vi "GenerateNewTag.vi"(8 "TagMarkerDuration (pws)":i32, 11 "Tag num":u32) -> (3 "digital waveform":digitalwaveform(waveform))   [LabVIEW 2017]
uses:
  <vilib>/Waveform/DWDTOps.llb/DWDT Boolean Array to Digital.vi
panel:
  out "Error Out":errorcluster
  in  "Error in":errorcluster
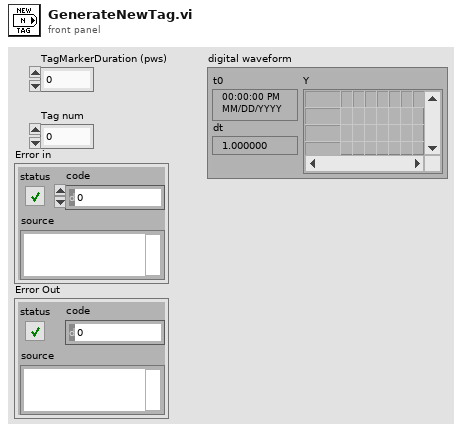
[diagram p1: front panel]
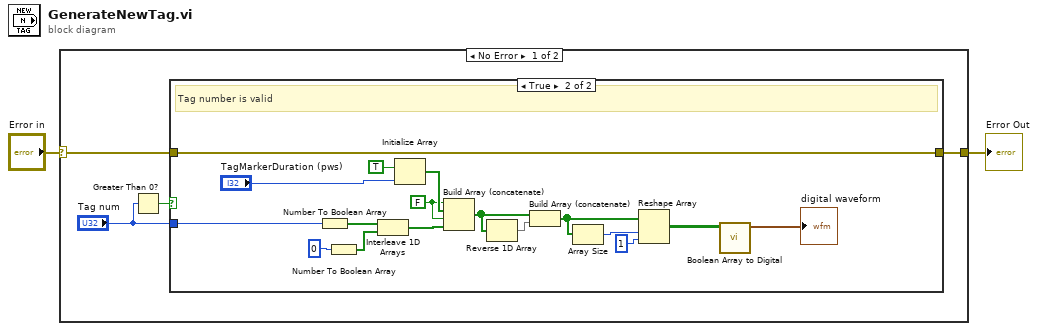
[diagram p0: block diagram]
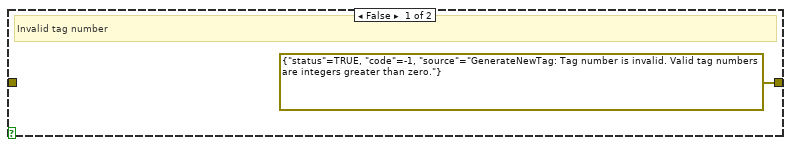
[diagram p2: hidden frame]
diagram:
  n1 = case shown="No Error" "Error in" {
    selector: "Error in" -> [w5 w25]
    tunnel: [w6 w25] -> w1
    frame No Error {
      n2 = Greater Than 0?(x="Tag num") -> (x > 0?=w3:bool)
      n3 = case shown="True" w3 {
        tunnel: [errorcluster {"status"=TRUE, "code"=-1, "source"="GenerateNewTag: Tag number is invalid. Valid tag numbers are integers greater than zero."} ("error IO") w16] -> w6
        tunnel: w5 -> [_ w16]
        tunnel: "Tag num" -> [_ w14]
        frame False {
          # "Invalid tag number"
        }
        frame True {
          w21 = FALSE ("Marker on")
          # "Tag number is valid"
          n4 = Number To Boolean Array(number=w14) -> (Boolean array=w18:bool[])
          n5 = Number To Boolean Array(number=0) -> (Boolean array=w19:bool[])
          n6 = Interleave 1D Arrays(w18, w19) -> (w20:bool[])
          n7 = Initialize Array(TRUE ("Marker on"), "TagMarkerDuration (pws)") -> (w23:bool[])
          n8 = Build Array (concatenate)(w21, w23, w21, w20) -> (w15:bool[])
          n9 = Reverse 1D Array(array=w15) -> (reversed array=w8:bool[])
          n10 = Build Array (concatenate)(w15, w8) -> (w13:bool[])
          n11 = Array Size(array=w13) -> (size(s)=w12:i32)
          n12 = Reshape Array(w13, w12, 1 ("dimension size")) -> (w11:bool[][])
          n13 = call-poly <vilib>:"Boolean Array to Digital.vi"("boolean array"=w11) -> ("digital waveform"=→"digital waveform":digitalwaveform)  [unwired: 9 in, 1 out]
        }
      }
    }
    frame Error {
    }
  }
  "Error Out" <- w1
